vi "LINX - PmodSONOR.vi"() -> ()   [LabVIEW 2011]
doc: "PmodMAXSONOR\n\nThis example demonstrates how to read the relative light sensed by the PmodALS.\n\nInstructions:\n1. Select the COM Port associated with the LINX device\n2. Select the UART Channel that the Pmod is connected to.\n3. Click the Run Arrow."
uses:
  vi.lib/MakerHub/LINX/Public/Utilities/Open Serial.vi
  vi.lib/MakerHub/LINX/LMH-LINX.lvlib
  vi.lib/MakerHub/LINX/Public/Sensors/Pmods/MAXSONAR/PmodMAXSONAR.lvlib
panel:
  out "Waveform Chart":u32(graph)
  out "Distance (in)":u32
  in  "Stop Button":bool
  in  "UART Channel (0)":u8=1
  in  "Serial Port":refnum<visa-resource-name>="N/A"
  # "PmodMAXSONOR\n\nThis example demonstrates how to read the relative light sensed by the PmodALS.\n\nInstructions:\n1. Select the COM Port associated with the LINX device\n2. Select the UART Channel that the Pmod is connected to.\n3. Click the Run Arrow."
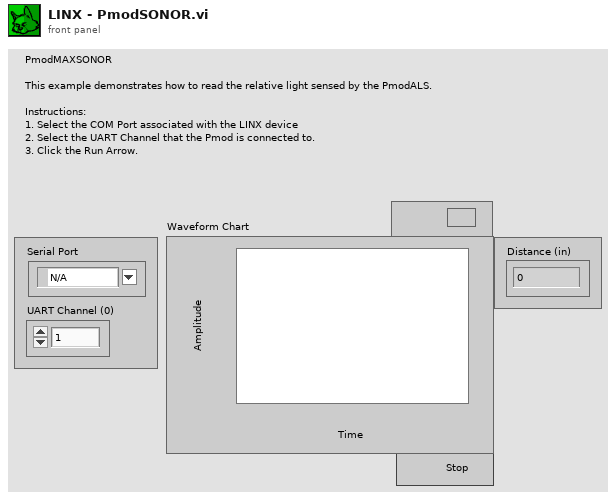
[diagram p1: front panel]
types:
  T1 = typedef "LMH-LINX.lvlib/LINX Ref.ctl" = cluster{"IO":T2, "Interface":T3, "LINX Device Config":T4}
  T2 = typedef "LMH-LINX.lvlib/Platform.ctl" = enum16{"Remote", "Local"}
  T3 = typedef "LMH-LINX.lvlib/Interface.ctl" = enum16{"Serial", "TCP"}
  T4 = typedef "LMH-LINX.lvlib/Device.lvlib/LINX Device Config.ctl" = cluster{"Interface":T3, "COM Port":refnum<visa-resource-name>, "TCP Configuration":T5, "Device Family":u8, "Device ID":u8, "Device Name":string, "TCP Ref":refnum<k5>, "Channels":T6}
  T5 = typedef "LMH-LINX.lvlib/Device.lvlib/TCP Config.ctl" = cluster{"IP Address":string, "Port":u16}
  T6 = typedef "LMH-LINX.lvlib/Channels.ctl" = cluster{"DI":u8[], "DO":u8[], "AI":u8[], "AO":u8[], "PWM":u8[], "QE":u8[], "UART":u8[], "I2C 2":u8[], "SPI":u8[], "CAN":u8[], "Servo":u8[], "AI Ref (V)":dbl, "AI Resolution (Bits)":u8, "AO Ref (V)":dbl, "AO Resolution (Bits)":u8}
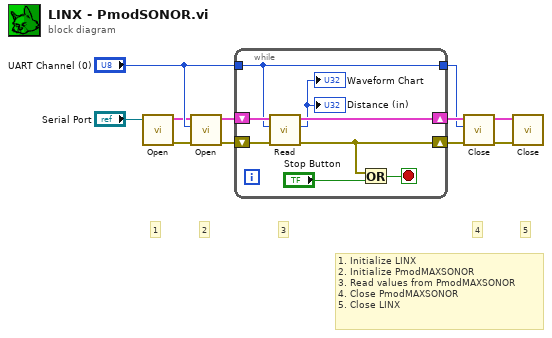
[diagram p0: block diagram]
diagram:
  # "1. Initialize LINX\n2. Initialize PmodMAXSONOR\n3. Read values from PmodMAXSONOR\n4. Close PmodMAXSONOR\n5. Close LINX"
  # "5"
  # "4"
  # "3"
  # "2"
  # "1"
  n1 = call-poly "Open.vi"("Serial Port"="Serial Port") -> ("Error Out"=w10:errorcluster, "LINX Resource"=w3:T1)  [unwired: 8 in, 1 out]
  n2 = call "Open.vi"("Error In"=w10, "UART Channel (0)"="UART Channel (0)", "LINX Resource"=w3) -> ("Error Out"=w7:errorcluster, "LINX Resource"=w6:T1)  [unwired: 7 in]
  n3 = while {
    shift-right: [w16] -> w5
    shift-left: w7 -> [w19]
    shift-right: [w14] -> w2
    shift-left: w6 -> [w15]
    tunnel: "UART Channel (0)" -> [w13]
    tunnel: [w13] -> w1
    stop <- w18 stop-if-true
    n4 = call "Read.vi"("Error In"=w19, "UART Channel (0)"=w13, "LINX Resource"=w15) -> ("Error Out"=w16:errorcluster, "Distance (in)"=→"Distance (in)" →"Waveform Chart":u32, "LINX Resource"=w14:T1)  [unwired: 6 in]
    n5 = Or(x=w16, y="Stop Button") -> (x .or. y?=w18:bool)
  }
  n6 = call "Close.vi"("Error In"=w5, "UART Channel (0)"=w1, "LINX Resource"=w2) -> ("Error Out"=w9:errorcluster, "LINX Resource"=w8:T1)  [unwired: 7 in]
  n7 = call "Close.vi"("Error In"=w9, "LINX Resource"=w8) -> ()  [unwired: 9 in, 1 out]
